vi "FileIO-Line to Array.vi"(0 "refnum":refnum<file>, 2 "Prefix":string, 11 "error in (no error)":errorcluster) -> (4 "refnum out":refnum<file>, 8 "array":dbl[](array[numeric]), 15 "error out":errorcluster)   [LabVIEW 2015]
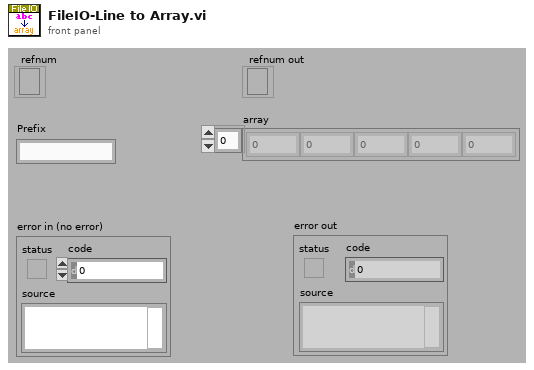
[diagram p1: front panel]
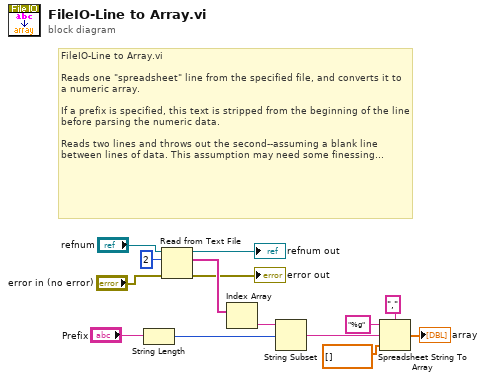
[diagram p0: block diagram]
diagram:
  # "FileIO-Line to Array.vi\n\nReads one \"spreadsheet\" line from the specified file, and converts it to a numeric array. \n\nIf a prefix is specified, this text is stripped from the beginning of the line before parsing the numeric data.\n\nReads two lines and throws out the second--assuming a blank line between lines of data. This assumption may need some finessing..."
  n1 = String Length(string="Prefix") -> (length=w3:i32)
  n2 = Read from Text File(file (use dialog)="refnum", count=2, error in="error in (no error)") -> (refnum out=→"refnum out":refnum<file>, text=w10:string[], error out=→"error out":errorcluster)  [unwired: 1 in, 1 out]
  n3 = Index Array(array=w10) -> (element=w7:string)  [unwired: 1 in]
  n4 = String Subset(string=w7, offset (0)=w3) -> (substring=w2:string)  [unwired: 1 in]
  n5 = Spreadsheet String To Array(delimiter (Tab)=",", format string="%g", spreadsheet string=w2, array type (2D Dbl)=dbl[] []) -> (array=→"array":dbl[])
